vi "Ocean Optics 2000 4000 Log Spectrum.vi"() -> ()   [LabVIEW 2021]
doc: "Demonstrates reading the spectra from the instrument and logging it in Excel file."
uses:
  <vilib>/Utility/file.llb/Write To Spreadsheet File (string).vi
  <vilib>/Utility/file.llb/Write To Spreadsheet File (DBL).vi
  <instrlib>/Ocean Optics 2000 4000/Ocean Optics 2000 4000.lvlib
panel:
  out "Log Data":dbl[][](array[numeric])
  in  "Number of Spectrum (5)":i32=5
  in  "VISA resource name":refnum<visa-resource-name>
  # "(c) 2009-2016 National Instruments.  ALL RIGHTS RESERVED."
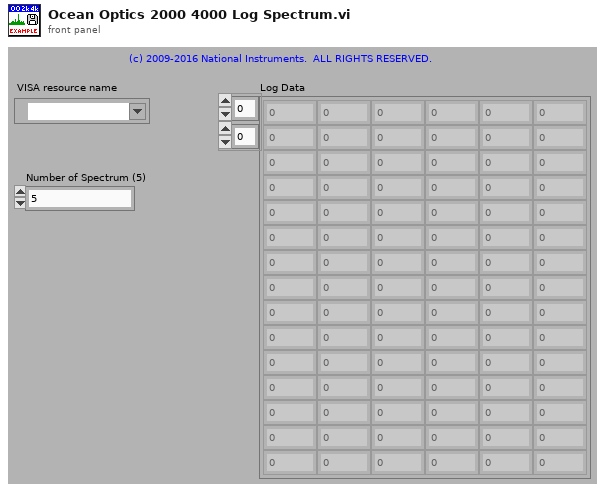
[diagram p1: front panel]
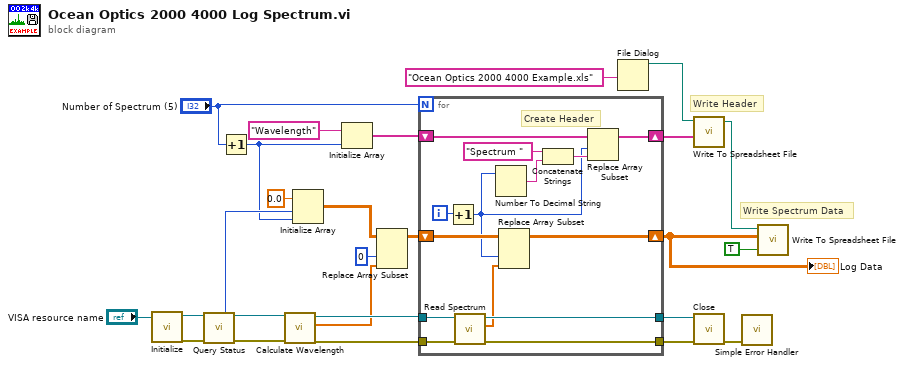
[diagram p0: block diagram]
diagram:
  # "Write Spectrum Data"
  # "Write Header"
  n1 = call <instrlib>:"Initialize.vi"("VISA resource name"="VISA resource name") -> ("error out"=w24:errorcluster, "VISA resource name out"=w25:refnum<visa-resource-name>)  [unwired: 2 in, 7 out]
  n2 = call <instrlib>:"Query Status.vi"("VISA resource name"=w25, "error in (no error)"=w24) -> ("Number of Pixels"=w10:u16, "VISA resource name out"=w23:refnum<visa-resource-name>, "error out"=w22:errorcluster)  [unwired: 11 out]
  n3 = Increment(x="Number of Spectrum (5)") -> (x+1=w7:i32)
  n4 = call <instrlib>:"Calculate Wavelength.vi"("error in (no error)"=w22, "VISA resource name"=w23) -> ("error out"=w20:errorcluster, "Wavelength (nm)"=w9:dbl[], "VISA resource name out"=w21:refnum<visa-resource-name>)  [unwired: 1 in, 6 out]
  n5 = Initialize Array(0.0 ("element"), w10, w7) -> (w17:dbl[][])
  n6 = Initialize Array("Wavelength", w7) -> (w6:string[])
  n7 = Replace Array Subset(array=w17, new element=w9, index (col)=0 ("disabled index (col)")) -> (w15:dbl[][])  [unwired: 1 in]
  n8 = for {
    N: "Number of Spectrum (5)" -> [_]
    tunnel: w21 -> [w40]
    tunnel: w20 -> [w39]
    tunnel: [w38] -> w4
    tunnel: [w37] -> w3
    shift-right: [w35] -> w1
    shift-left: w15 -> [w36]
    shift-right: [w28] -> w5
    shift-left: w6 -> [w31]
    i -> [w27]
    # "Create Header"
    n9 = Increment(x=w27) -> (x+1=w29:i32)
    n10 = call <instrlib>:"Read Spectrum.vi"("error in (no error)"=w39, "VISA resource name"=w40) -> ("error out"=w37:errorcluster, "Spectrum by Pixel Number"=w34:dbl[], "VISA resource name out"=w38:refnum<visa-resource-name>)  [unwired: 6 in, 1 out]
    n11 = Number To Decimal String(number=w29) -> (decimal integer string=w33:string)  [unwired: 1 out]
    n12 = Replace Array Subset(array=w36, new element=w34, index (col)=w29) -> (w35:dbl[][])  [unwired: 1 in]
    n13 = Concatenate Strings("Spectrum " ("string"), w33) -> (w30:string)
    n14 = Replace Array Subset(array=w31, new element=w30, index=w29) -> (w28:string[])
  }
  "Log Data" <- w1
  n15 = File Dialog(9:"Ocean Optics 2000 4000 Example.xls" ("default name")) -> (3:w13:path)  [unwired: 1 in, 8 out]
  n16 = call-poly <vilib>:"Write To Spreadsheet File.vi"("1D data"=w5, "file path (dialog if empty)"=w13) -> ("new file path (Not A Path if cancelled)"=w12:path)  [unwired: 4 in, 2 out]
  n17 = call <instrlib>:"Close.vi"("error in (no error)"=w3, "VISA resource name"=w4) -> ("error out"=w2:errorcluster)  [unwired: 9 out]
  n18 = call <vilib>:"Simple Error Handler.vi"("error in (no error)"=w2) -> ()  [unwired: 1 in, 8 out]
  n19 = call-poly <vilib>:"Write To Spreadsheet File.vi"("append to file? (new file:F)"=TRUE, "2D data"=w1, "file path (dialog if empty)"=w12) -> ()  [unwired: 3 in, 3 out]
